vi "TwDaqActive.vi"() -> (0 "DAQ active?":bool)   [LabVIEW 2009]
uses:
  TofDaqDll.dll
panel:
  in  "error in (no error)":errorcluster
  out "error out":errorcluster
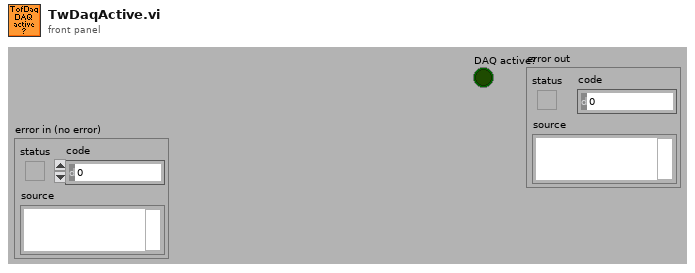
[diagram p1: front panel]
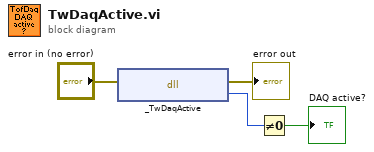
[diagram p0: block diagram]
diagram:
  n1 = dll-call lib="C:/Users/TofEmp/Desktop/LVTest/TofDaqDll.dll" fn="_TwDaqActive"(error in="error in (no error)") -> (error out=→"error out":errorcluster, "return type"=w2:i8)  [unwired: 2 in, 1 out]
  n2 = Not Equal To 0?(x=w2) -> (x != 0?=→"DAQ active?":bool)
